vi "alignment_main.vi"() -> ()   [LabVIEW 2011]
uses:
  <vilib>/userdefined/High Color/IMAQdx.ctl
  global_vars.vi
  <vilib>/vision/driver/NI_Vision_Acquisition_Software.lvlib
  C:/Program Files/National Instruments/LabVIEW 2011/resource/objmgr/imaqdx.rc
panel:
  in  "stream_overlay":bool
  in  "save":bool
  in  "File Path":path
  in  "Shutter Speed":dbl(slide)=1e-10 min=1e-10 max=1.0 scale=0.0..0.25
  out "Image":T1(plugin-control)
  in  "flip direction":bool
  in  "stream_OL_center_radius":dbl
  in  "stream_OL_#rings":i32
  in  "df_intial phase shift":dbl
  in  "df_#fringes":dbl=4.0 caption="#fringes"
  in  "fringe_OL_#rings":i32=20
  in  "fringe_OL_center_radius":dbl
  in  "fringe_OL_color":u32(colorbox)=16448250
  in  "b_align":bool=TRUE
  in  "b_preview fringes":bool
  in  "fullscreen?":bool
  in  "y height(Px)":i32=500
  in  "x Width(Px)":i32=1000
  in  "to second \nscreen?":bool
  in  "floating":bool=TRUE
  in  "title bar":bool=TRUE
  in  "stream_OL_color":u32(colorbox)=16448250
  in  "Close":bool
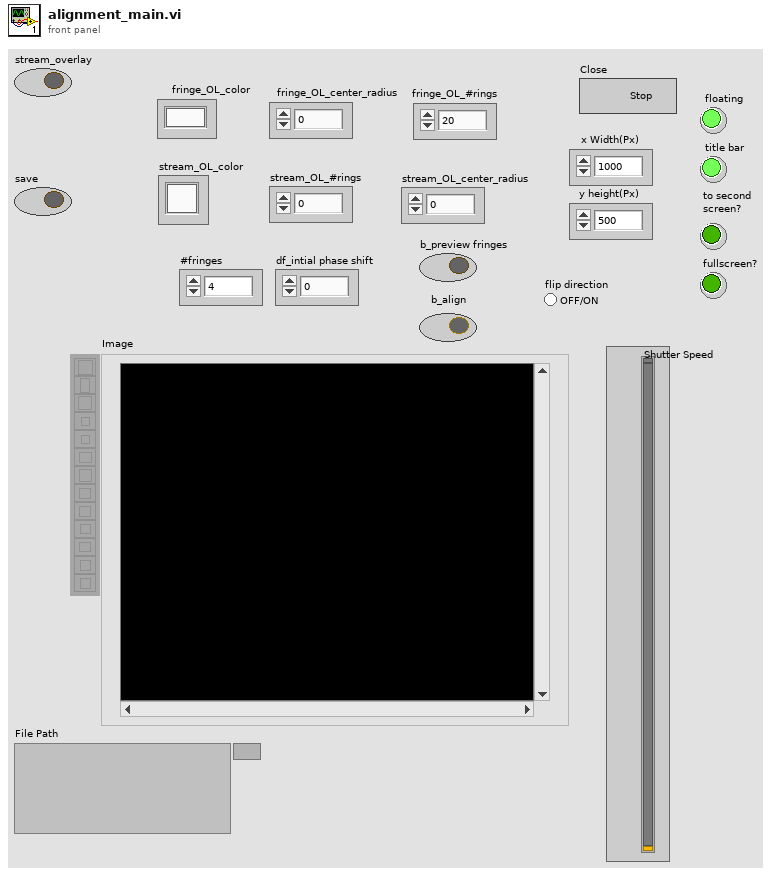
[diagram p1: front panel]
types:
  T1 = typedef "IMAQ Image.ctl" = refnum<image>
  T2 = enum8{"Enabled", "Disabled", "Disabled and Grayed Out"}
  T3 = typedef "IMAQdx.ctl" = refnum<k21>
  T4 = cluster{"Numeric Control":i16, "Numeric Control":i16}
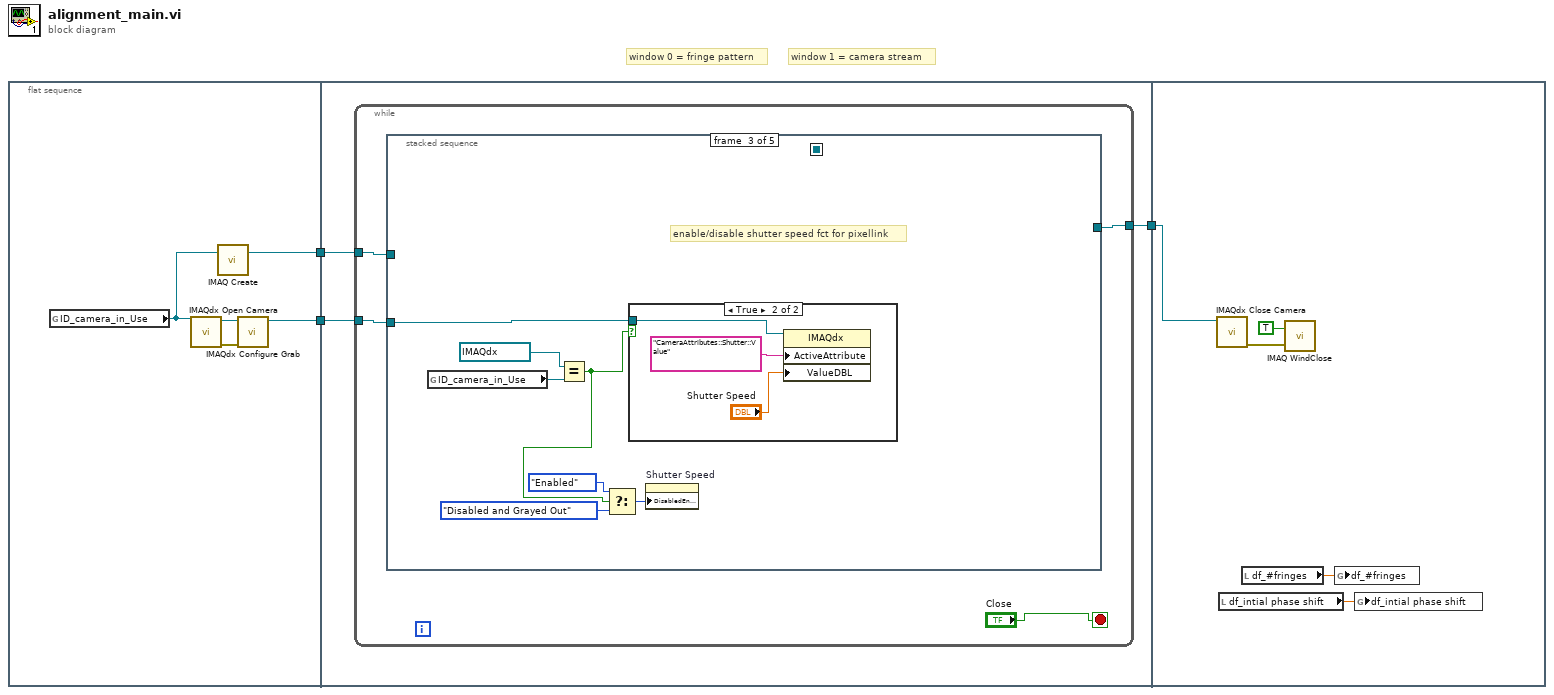
[diagram p0: block diagram]
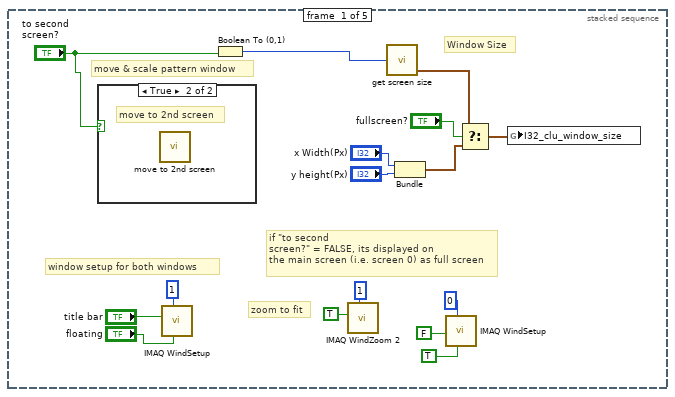
[diagram p2: hidden frame]
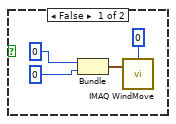
[diagram p3: hidden frame]
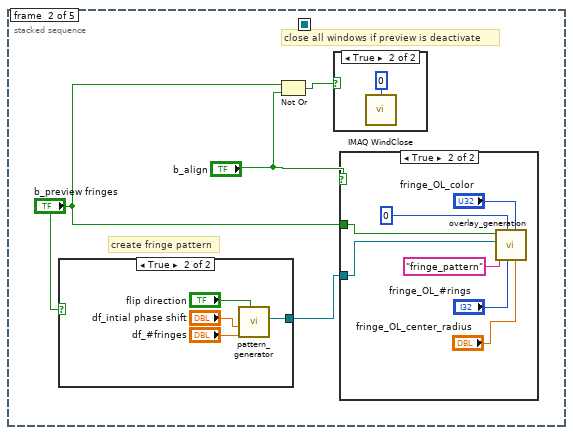
[diagram p4: hidden frame]
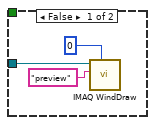
[diagram p6: hidden frame]
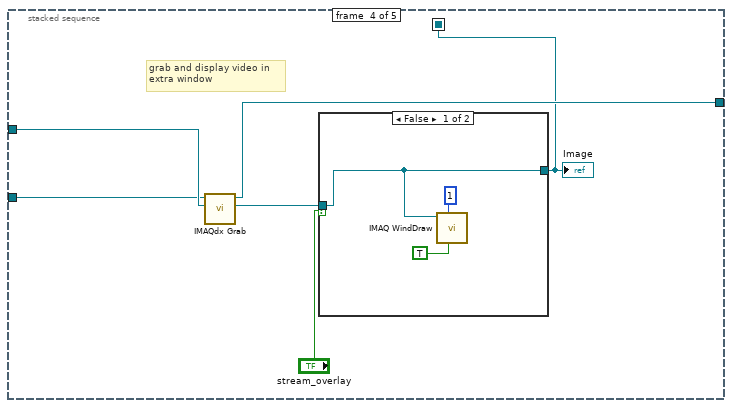
[diagram p9: hidden frame]
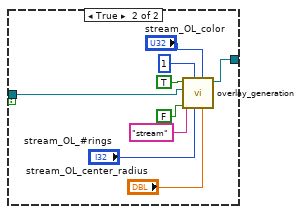
[diagram p10: hidden frame]
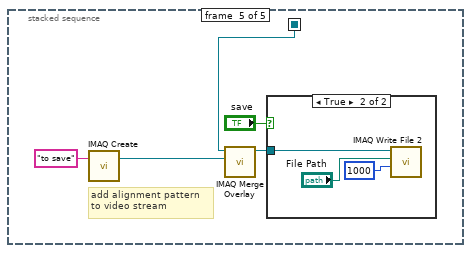
[diagram p11: hidden frame]
diagram:
  # "window 1 = camera stream"
  # "window 0 = fringe pattern"
  n1 = flat-sequence {
    tunnel: [w4] -> w2
    tunnel: [w5] -> w1
    tunnel: [w9] -> w3
    tunnel: w2 -> [w11]
    tunnel: w1 -> [w10]
    tunnel: w3 -> [w91]
    frame #0 {
      n2 = global read "global_vars.vi" "ID_camera_in_Use"() -> (w8:T3)
      n3 = call <vilib>:"IMAQdx Open Camera.vi"("Session In"=w8) -> ("error out"=w6:errorcluster, "Session Out"=w7:T3)  [unwired: 2 in, 7 out]
      n4 = call "IMAQ Create"("Image Name"=w8) -> ("New Image"=w4:T1)  [unwired: 3 in, 2 out]
      n5 = call <vilib>:"IMAQdx Configure Grab.vi"("error in"=w6, "Session In"=w7) -> ("Session Out"=w5:T3)  [unwired: 9 out]
    }
    frame #1 {
      n6 = while {
        tunnel: w10 -> [w15]
        tunnel: w11 -> [w14]
        tunnel: [w12] -> w9
        stop <- "Close" stop-if-true
        n7 = stacked-sequence {
          seq-local: [_ _ _ w66 _] -> [_ _ _ _ w83]
          tunnel: w15 -> [_ _ w55 w68 _]
          tunnel: w14 -> [_ _ _ w70 _]
          tunnel: [_ _ _ w69 _] -> w12
          frame #0 {
            # "zoom to fit"
            # "if \"to second \nscreen?\" = FALSE, its displayed on \nthe main screen (i.e. screen 0) as full screen"
            # "window setup for both windows"
            # "Window Size"
            # "move & scale pattern window"
            n8 = case shown="True" "to second \nscreen?" {
              frame False {
                n9 = Bundle(0, 0) -> (w35:cluster{i32, i32})  [unwired: 1 in]
                n10 = call "IMAQ WindMove"("Window Number (0...15)"=0, "Coordinates (screen)"=w35) -> ()  [unwired: 3 in, 2 out]
              }
              frame True {
                # "move to 2nd screen"
                n11 = call "move to 2nd screen.vi"() -> ()  [unwired: 12 in]
              }
            }
            n12 = call "IMAQ WindSetup"("Window is floating? (No)"="floating", "Window Number (0...15)"=1, "Window has title bar? (Yes)"="title bar") -> ()  [unwired: 8 in, 1 out]
            n13 = Boolean To (0,1)(Boolean="to second \nscreen?") -> (0, 1=w31:i16)
            n14 = call "IMAQ WindZoom 2"("Window Number (0...15)"=1, "Zoom to Fit? (False)"=TRUE) -> ()  [unwired: 6 in, 4 out]
            n15 = call "get screen size.vi"("screen"=w31) -> ("wind size (width/height)"=w30:T4)  [unwired: 2 in, 2 out]
            n16 = Bundle("x Width(Px)"="x Width(Px)", "y height(Px)"="y height(Px)") -> (w28:cluster{"x Width(Px)":i32, "y height(Px)":i32})  [unwired: 1 in]
            n17 = call "IMAQ WindSetup"("Window is floating? (No)"=TRUE, "Window Number (0...15)"=0, "Window has title bar? (Yes)"=FALSE) -> ()  [unwired: 8 in, 1 out]
            n18 = Select(t=w30, s="fullscreen?", f=w28) -> (s? t:f=w29:cluster{"x Width(Px)":i32, "y height(Px)":i32})
            n19 = global write "global_vars.vi" "I32_clu_window_size"(w29) -> ()
          }
          frame #1 {
            # "close all windows if preview is deactivate"
            # "create fringe pattern"
            n20 = case shown="True" "b_preview fringes" {
              tunnel: [_ w54] -> w36
              frame False {
              }
              frame True {
                n21 = call "pattern_generator.vi"("flip direction"="flip direction", "fringe number"="df_#fringes", "phase"="df_intial phase shift") -> ("fringe pattern"=w54:T1)  [unwired: 7 in, 1 out]
              }
            }
            n22 = Not Or(1:"b_align", 2:"b_preview fringes") -> (0:w37:bool)
            n23 = case shown="True" w37 {
              frame False {
              }
              frame True {
                n24 = call "IMAQ WindClose"("Window Number (0...15)"=0) -> ()  [unwired: 5 in, 1 out]
              }
            }
            n25 = case shown="True" "b_align" {
              tunnel: w36 -> [w42 w50]
              tunnel: "b_preview fringes" -> [_ w49]
              frame False {
                n26 = call "IMAQ WindDraw"("Window Number (0...15)"=0, "Title"="preview", "Image"=w42) -> ()  [unwired: 7 in, 2 out]
              }
              frame True {
                n27 = call "overlay_generation.vi"("center radius"="fringe_OL_center_radius", "Color"="fringe_OL_color", "number of rings"="fringe_OL_#rings", "Window Number (0...15)"=0, "Title"="fringe_pattern", "Image Src"=w50, "fringe preview on"=w49) -> ()  [unwired: 4 in, 1 out]
              }
            }
          }
          frame #2 {
            # "enable/disable shutter speed fct for pixellink"
            n28 = global read "global_vars.vi" "ID_camera_in_Use"() -> (w60:T3)
            n29 = Equal?(x=T3 "PixeLink" ("ID_camera_in_Use"), y=w60) -> (x = y?=w59:bool)
            n30 = Select(t=T2."Enabled" ("Disabled"), s=w59, f=T2."Disabled and Grayed Out" ("Disabled")) -> (s? t:f=w56:T2)
            n31 = case shown="True" w59 {
              tunnel: w55 -> [_ w62]
              frame False {
              }
              frame True {
                n32 = property class="IMAQdx"(reference=w62, "ActiveAttribute"="CameraAttributes::Shutter::Value", "ValueDBL"="Shutter Speed") -> ()  [unwired: 1 in, 2 out]
              }
            }
            n33 = property on="Shutter Speed" class="Slide (strict)"("DisabledEnum"=w56) -> ()  [unwired: 2 in, 2 out]
          }
          frame #3 {
            # "grab and display video in \nextra window"
            n34 = call <vilib>:"IMAQdx Grab.vi"("Image In"=w70, "Session In"=w68) -> ("Image Out"=w67:T1, "Session Out"=w69:T3)  [unwired: 2 in, 6 out]
            n35 = case shown="False" "stream_overlay" {
              tunnel: w67 -> [w73 w75]
              tunnel: [w73 w74] -> w66
              frame False {
                n36 = call "IMAQ WindDraw"("Resize to Image Size? (Y)"=TRUE, "Window Number (0...15)"=1, "Image"=w73) -> ()  [unwired: 7 in, 2 out]
              }
              frame True {
                n37 = call "overlay_generation.vi"("center radius"="stream_OL_center_radius", "Color"="stream_OL_color", "number of rings"="stream_OL_#rings", "Window Number (0...15)"=1, "Resize to Image Size? (Y)"=FALSE, "Title"="stream", "Image Src"=w75, "fringe preview on"=TRUE) -> ("stream_overlay_out"=w74:T1)  [unwired: 3 in]
              }
            }
            "Image" <- w66
          }
          frame #4 {
            # "add alignment pattern \nto video stream"
            n38 = call "IMAQ Create"("Image Name"="to save") -> ("New Image"=w84:T1)  [unwired: 3 in, 2 out]
            n39 = call "IMAQ Merge Overlay"("Image Dst"=w84, "Image Src"=w83) -> ("Image Dst Out"=w86:T1)  [unwired: 8 in, 1 out]
            n40 = case shown="True" "save" {
              tunnel: w86 -> [_ w90]
              frame False {
              }
              frame True {
                n41 = call-poly "IMAQ Write File 2"("Image Quality"=u32 1000, "File Path"="File Path", "Image"=w90) -> ()  [unwired: 7 in, 2 out]
              }
            }
          }
        }
      }
    }
    frame #2 {
      n42 = call <vilib>:"IMAQdx Close Camera.vi"("Session In"=w91) -> ("error out"=w93:errorcluster)  [unwired: 1 in, 9 out]
      n43 = local read "df_intial phase shift"() -> (w95:dbl)
      n44 = local read "df_#fringes"() -> (w94:dbl)
      n45 = call "IMAQ WindClose"("Close All Windows (False)"=TRUE, "error in (no error)"=w93) -> ()  [unwired: 4 in, 1 out]
      n46 = global write "global_vars.vi" "df_#fringes"(w94) -> ()
      n47 = global write "global_vars.vi" "df_intial phase shift"(w95) -> ()
    }
  }
